vi "Write Client types.vi"(8 "error in (no error)":errorcluster, 10 "Client types":string[](array[string]), 11 "Get-clients in":refnum<class "Get-clients.lvclass">) -> (0 "error out":errorcluster, 3 "Get-clients out":refnum<class "Get-clients.lvclass">)   [LabVIEW 2013, in "SLMAPI.lvlib" / "Get-clients.lvclass"]
uses:
  Get-clients.lvclass
  Get-clients.lvclass/Get-clients.ctl
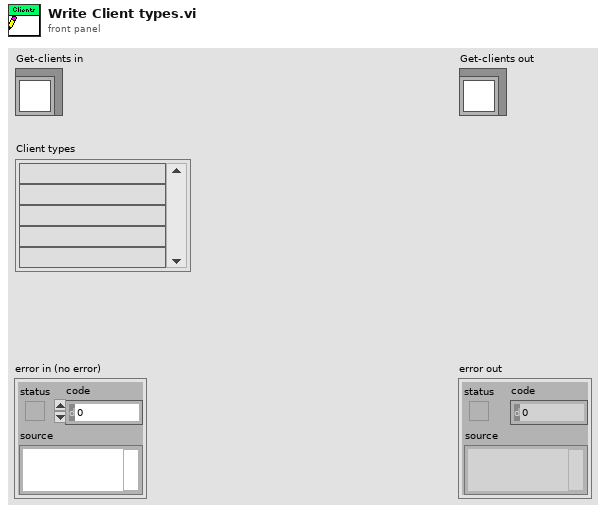
[diagram p1: front panel]
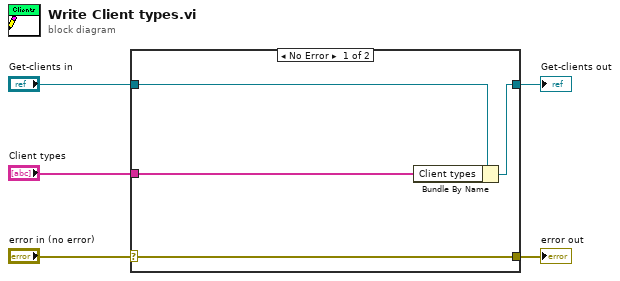
[diagram p0: block diagram]
diagram:
  n1 = case shown="No Error" "error in (no error)" {
    selector: "error in (no error)" -> [w9 w10]
    tunnel: [w9 w10] -> w4
    tunnel: [w7 w11] -> w2
    tunnel: "Get-clients in" -> [w8 w11]
    tunnel: "Client types" -> [w6 _]
    frame No Error {
      n2 = Bundle By Name(cluster=w8, "Client types"=w6) -> (w7:refnum<class "Get-clients.lvclass">)
    }
    frame Error {
    }
  }
  "error out" <- w4
  "Get-clients out" <- w2
